vi "Check Escala.vi"(8 "error in (no error)":errorcluster, 10 "Grandeza":string, 11 "TY720 in":refnum<class "TY720.lvclass">) -> (0 "error out":errorcluster, 2 "Escala Correta?":bool, 3 "TY720 out":refnum<class "TY720.lvclass">)   [LabVIEW 2015, in "TY720.lvclass"]
uses:
  TY720.lvclass
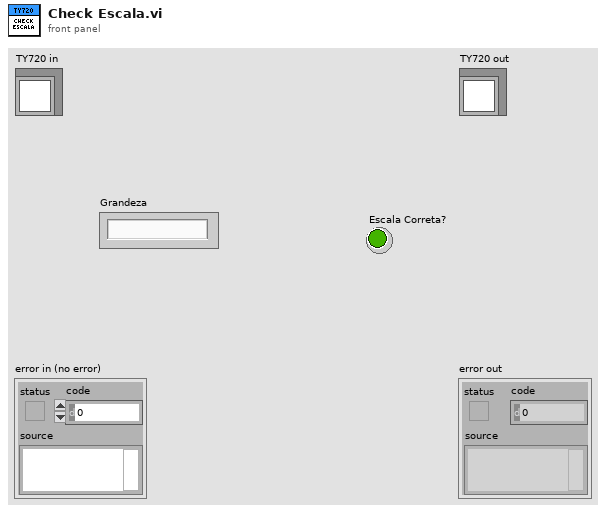
[diagram p1: front panel]
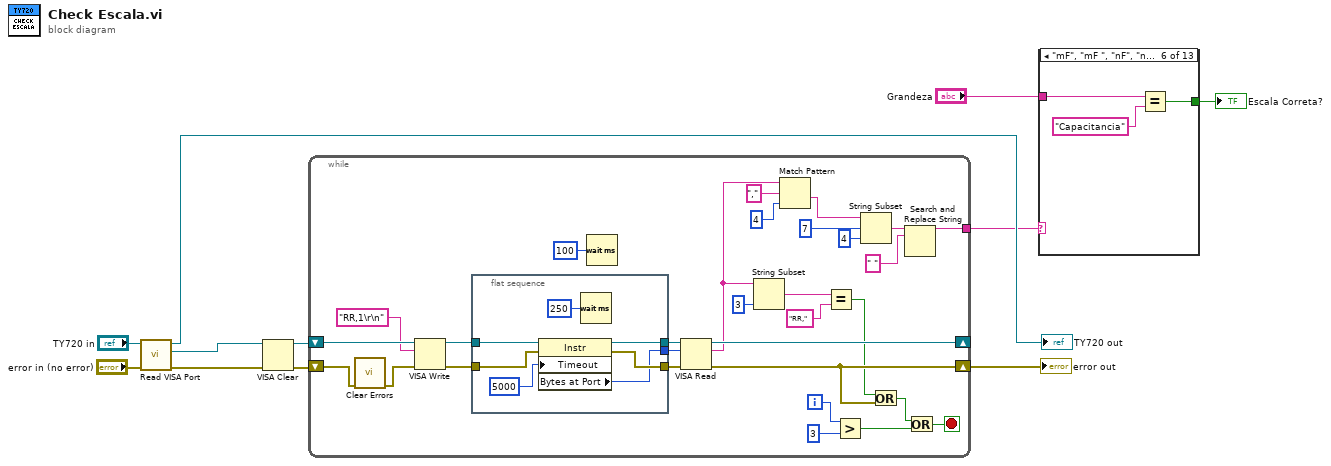
[diagram p0: block diagram]
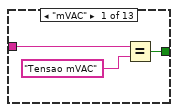
[diagram p2: hidden frame]
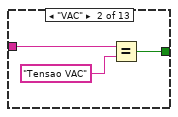
[diagram p3: hidden frame]
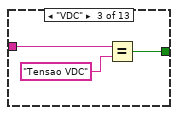
[diagram p4: hidden frame]
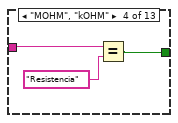
[diagram p5: hidden frame]
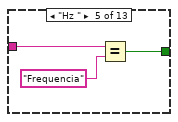
[diagram p6: hidden frame]
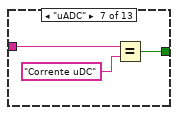
[diagram p7: hidden frame]
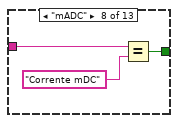
[diagram p8: hidden frame]
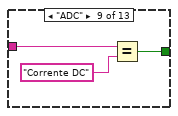
[diagram p9: hidden frame]
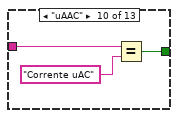
[diagram p10: hidden frame]
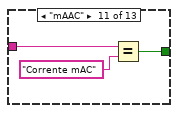
[diagram p11: hidden frame]
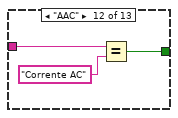
[diagram p12: hidden frame]
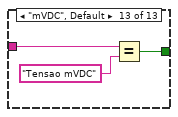
[diagram p13: hidden frame]
diagram:
  n1 = call-dynamic "Read VISA Port.vi"("error in (no error)"="error in (no error)", "Device in"="TY720 in") -> ("error out"=w9:errorcluster, "VISA Port"=w1:refnum<visa-resource-name>, "Device out"=→"TY720 out":refnum<class "TY720.lvclass">)  [unwired: 7 in]
  n2 = VISA Clear(VISA resource name=w1, error in (no error)=w9) -> (VISA resource name out=w10:refnum<visa-resource-name>, error out=w11:errorcluster)
  n3 = while {
    shift-right: [w26] -> w5
    shift-left: w11 -> [w32]
    shift-right: [w40] -> _
    shift-left: w10 -> [w41]
    tunnel: [w12] -> w3
    i -> [w34]
    stop <- w27 stop-if-true
    n4 = call <vilib>:"Clear Errors.vi"("error in (no error)"=w32) -> ("error out"=w31:errorcluster)  [unwired: 5 in, 1 out]
    n5 = VISA Write(VISA resource name=w41, write buffer="RR,1\r\n", error in (no error)=w31) -> (VISA resource name out=w38:refnum<visa-resource-name>, error out=w36:errorcluster)  [unwired: 1 out]
    n6 = flat-sequence {
      tunnel: w38 -> [w48]
      tunnel: [w46] -> w37
      tunnel: w36 -> [w45]
      tunnel: [w44] -> w35
      tunnel: [w43] -> w24
      frame #0 {
        n7 = property class="Instr"(reference=w48, error in=w45, "Timeout"=u32 5000 ("General Settings:Timeout Value")) -> (reference out=w46:refnum<visa-resource-name>, error out=w44:errorcluster, "Bytes at Port"=w43:u32)
        n8 = Wait (ms)(milliseconds to wait=u32 250) -> ()  [unwired: 1 out]
      }
    }
    n9 = Wait (ms)(milliseconds to wait=u32 100) -> ()  [unwired: 1 out]
    n10 = VISA Read(VISA resource name=w37, byte count=w24, error in (no error)=w35) -> (VISA resource name out=w40:refnum<visa-resource-name>, read buffer=w20:string, error out=w26:errorcluster)  [unwired: 1 out]
    n11 = String Subset(string=w20, length (rest)=3 ("length (rest)")) -> (substring=w21:string)  [unwired: 1 in]
    n12 = Match Pattern(string=w20, regular expression=",", offset (0)=4) -> (after substring=w17:string)  [unwired: 3 out]
    n13 = Equal?(x=w21, y="RR,") -> (x = y?=w23:bool)
    n14 = Greater?(x=w34, y=3) -> (0:w28:bool)
    n15 = String Subset(string=w17, offset (0)=7, length (rest)=4 ("length (rest)")) -> (substring=w13:string)
    n16 = Or(x=w23, y=w26) -> (x .or. y?=w25:bool)
    n17 = Search and Replace String(input string=w13, search string=" ") -> (result string=w12:string)  [unwired: 6 in, 3 out]
    n18 = Or(x=w25, y=w28) -> (x .or. y?=w27:bool)
  }
  "error out" <- w5
  n19 = case shown="\"mF\", \"mF \", \"nF\", \"nF \", \"uF\", \"uF \"" w3 {
    tunnel: "Grandeza" -> [w51 w54 w57 w60 w63 w66 w69 w72 w75 w78 w81 w84 w85]
    tunnel: [w49 w52 w55 w59 w61 w65 w68 w71 w74 w77 w80 w83 w86] -> w2
    frame "mVAC" {
      n20 = Equal?(x=w51, y="Tensao mVAC") -> (x = y?=w49:bool)
    }
    frame "VAC" {
      n21 = Equal?(x=w54, y="Tensao VAC") -> (x = y?=w52:bool)
    }
    frame "VDC" {
      n22 = Equal?(x=w57, y="Tensao VDC") -> (x = y?=w55:bool)
    }
    frame "MOHM", "kOHM" {
      n23 = Equal?(x=w60, y="Resistencia") -> (x = y?=w59:bool)
    }
    frame "Hz " {
      n24 = Equal?(x=w63, y="Frequencia") -> (x = y?=w61:bool)
    }
    frame "mF", "mF ", "nF", "nF ", "uF", "uF " {
      n25 = Equal?(x=w66, y="Capacitancia") -> (x = y?=w65:bool)
    }
    frame "uADC" {
      n26 = Equal?(x=w69, y="Corrente uDC") -> (x = y?=w68:bool)
    }
    frame "mADC" {
      n27 = Equal?(x=w72, y="Corrente mDC") -> (x = y?=w71:bool)
    }
    frame "ADC" {
      n28 = Equal?(x=w75, y="Corrente DC") -> (x = y?=w74:bool)
    }
    frame "uAAC" {
      n29 = Equal?(x=w78, y="Corrente uAC") -> (x = y?=w77:bool)
    }
    frame "mAAC" {
      n30 = Equal?(x=w81, y="Corrente mAC") -> (x = y?=w80:bool)
    }
    frame "AAC" {
      n31 = Equal?(x=w84, y="Corrente AC") -> (x = y?=w83:bool)
    }
    frame "mVDC", Default {
      n32 = Equal?(x=w85, y="Tensao mVDC") -> (x = y?=w86:bool)
    }
  }
  "Escala Correta?" <- w2
